vi "test-twist3d.vi"(8 "error in (no error)":errorcluster) -> (0 "error out":errorcluster, 3 "All PASSED":bool)   [LabVIEW 2019]
uses:
  <vilib>/Rock Robotics/WPI/ThirdParty/JAS_Junk/TrajLib/Pose3d_New_Trans3dRot3d.vi
  <vilib>/Rock Robotics/WPI/ThirdParty/JAS_Junk/TrajLib/Translation3d_Create_Default.vi
  <vilib>/Rock Robotics/WPI/ThirdParty/JAS_Junk/TrajLib/Quaternion_New_Default.vi
  <vilib>/Rock Robotics/WPI/ThirdParty/JAS_Junk/TrajLib/Quaternion_New.vi
  <vilib>/Rock Robotics/WPI/ThirdParty/JAS_Junk/TrajLib/Translation3d_Create.vi
  <vilib>/Rock Robotics/WPI/ThirdParty/JAS_Junk/TrajLib/Translation3d_Equals.vi
  <vilib>/Rock Robotics/WPI/ThirdParty/JAS_Junk/TrajLib/Rotation3d_Equals.vi
  <vilib>/Rock Robotics/WPI/ThirdParty/JAS_Junk/TrajLib/Pose3d_getTranslation3d.vi
  <vilib>/Rock Robotics/WPI/ThirdParty/JAS_Junk/TrajLib/Pose3d_getRotation3d.vi
  <vilib>/Rock Robotics/WPI/ThirdParty/JAS_Junk/TrajLib/Matrix_NormF.vi
  <vilib>/Rock Robotics/WPI/ThirdParty/JAS_Junk/TrajLib/Rotation3d_GetQuaterion.vi
  <vilib>/Rock Robotics/WPI/ThirdParty/JAS_Junk/TrajLib/Quaternion_Equals.vi
  <vilib>/Analysis/_algsub.llb/Matrix Norm.vi
  <vilib>/Analysis/_algsub.llb/Real Matrix Norm.vi
  <vilib>/Analysis/Matrix/Numeric/Conversions/Array To Matrix.vi
  <vilib>/Analysis/Matrix/Numeric/Conversions/Array To Matrix - RA.vi
  <vilib>/Rock Robotics/WPI/ThirdParty/JAS_Junk/TrajLib/Trajectory_Library.lvlib
panel:
  # "Twist3d Test"
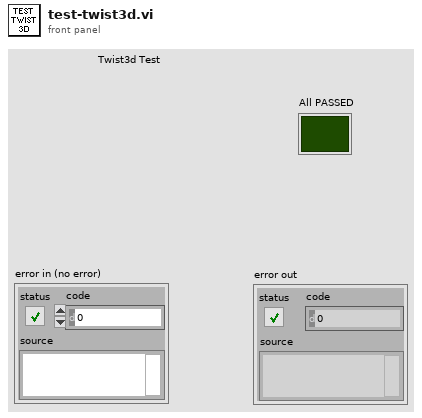
[diagram p1: front panel]
types:
  T1 = typedef "Trajectory_Library.lvlib/ROTATION3D.ctl" = cluster{"Q_quaternion":T2}
  T2 = typedef "Trajectory_Library.lvlib/QUATERNION.ctl" = cluster{"R":dbl, "V":dbl[]}
  T3 = typedef "Trajectory_Library.lvlib/POSE3D.ctl" = cluster{"Translation3d":T4, "Rotation3d":T1}
  T4 = typedef "Trajectory_Library.lvlib/TRANSLATION3D.ctl" = cluster{"X":dbl, "Y":dbl, "Z":dbl}
  T5 = typedef "Trajectory_Library.lvlib/TWIST3D.ctl" = cluster{"dX":dbl, "dY":dbl, "dZ":dbl, "rX":dbl, "rY":dbl, "rZ":dbl}
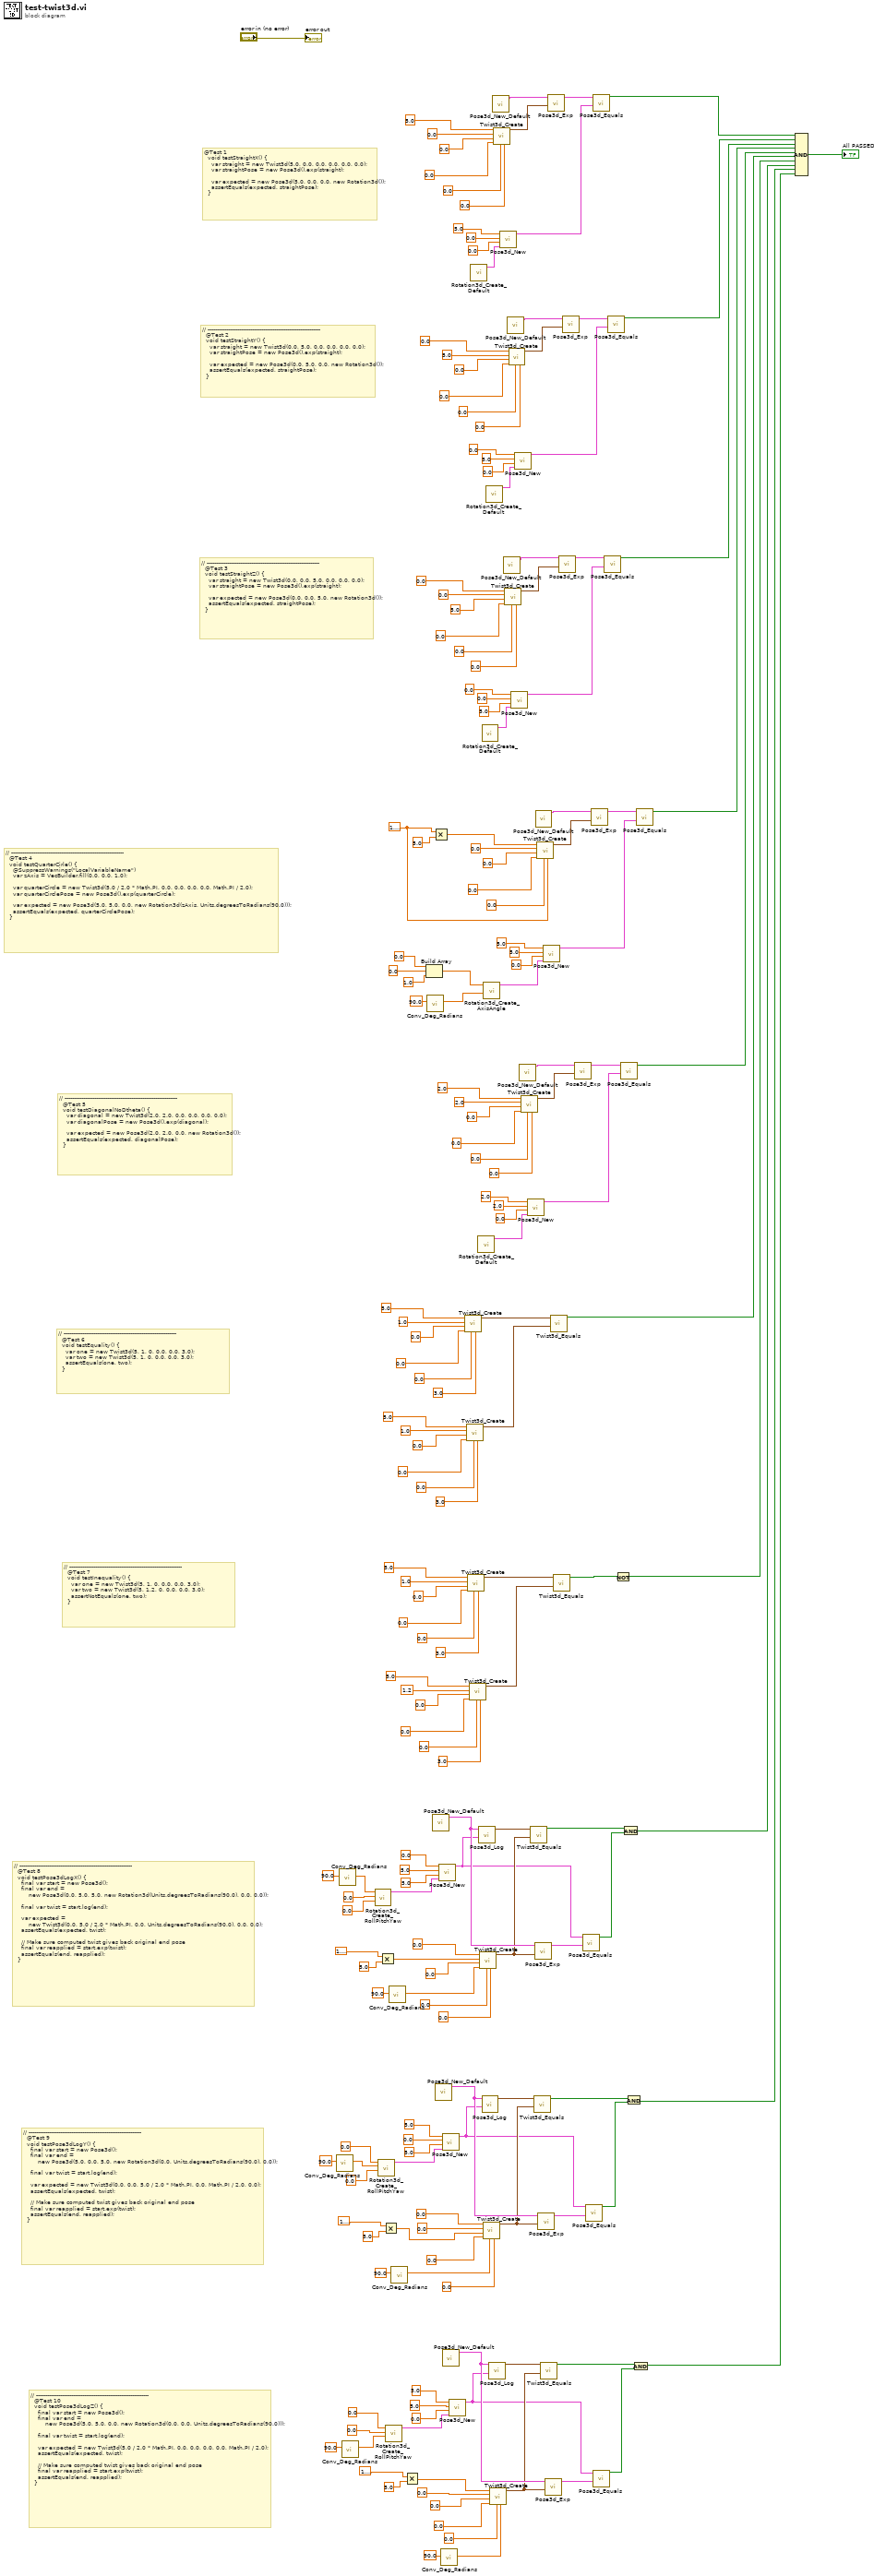
[diagram p0: block diagram]
diagram:
  w130 = 1.5707963267948966
  # "// -------------------------------------------------------------\n  @Test 10\n  void testPose3dLogZ() {\n    final var start = new Pose3d();\n    final var end =\n        new Pose3d(5.0, 5.0, 0.0, new Rotation3d(0.0, 0.0, Units.degreesToRadians(90.0)));\n\n    final var twist = start.log(end);\n\n    var expected = new Twist3d(5.0 / 2.0 * Math.PI, 0.0, 0.0, 0.0, 0.0, Math.PI / 2.0);\n    assertEquals(expected, twist);\n\n    // Make sure computed twist gives back original end pose\n    final var reapplied = start.exp(twist);\n    assertEquals(end, reapplied);\n  }"
  # "// -------------------------------------------------------------\n  @Test 9\n  void testPose3dLogY() {\n    final var start = new Pose3d();\n    final var end =\n        new Pose3d(5.0, 0.0, 5.0, new Rotation3d(0.0, Units.degreesToRadians(90.0), 0.0));\n\n    final var twist = start.log(end);\n\n    var expected = new Twist3d(0.0, 0.0, 5.0 / 2.0 * Math.PI, 0.0, Math.PI / 2.0, 0.0);\n    assertEquals(expected, twist);\n\n    // Make sure computed twist gives back original end pose\n    final var reapplied = start.exp(twist);\n    assertEquals(end, reapplied);\n  }"
  # "// -------------------------------------------------------------\n  @Test 8\n  void testPose3dLogX() {\n    final var start = new Pose3d();\n    final var end =\n        new Pose3d(0.0, 5.0, 5.0, new Rotation3d(Units.degreesToRadians(90.0), 0.0, 0.0));\n\n    final var twist = start.log(end);\n\n    var expected =\n        new Twist3d(0.0, 5.0 / 2.0 * Math.PI, 0.0, Units.degreesToRadians(90.0), 0.0, 0.0);\n    assertEquals(expected, twist);\n\n    // Make sure computed twist gives back original end pose\n    final var reapplied = start.exp(twist);\n    assertEquals(end, reapplied);\n  }"
  # "// -------------------------------------------------------------\n  @Test 7\n  void testInequality() {\n    var one = new Twist3d(5, 1, 0, 0.0, 0.0, 3.0);\n    var two = new Twist3d(5, 1.2, 0, 0.0, 0.0, 3.0);\n    assertNotEquals(one, two);\n  }"
  # "// -------------------------------------------------------------\n  @Test 6\n  void testEquality() {\n    var one = new Twist3d(5, 1, 0, 0.0, 0.0, 3.0);\n    var two = new Twist3d(5, 1, 0, 0.0, 0.0, 3.0);\n    assertEquals(one, two);\n  }"
  # "// -------------------------------------------------------------\n  @Test 5\n  void testDiagonalNoDtheta() {\n    var diagonal = new Twist3d(2.0, 2.0, 0.0, 0.0, 0.0, 0.0);\n    var diagonalPose = new Pose3d().exp(diagonal);\n\n    var expected = new Pose3d(2.0, 2.0, 0.0, new Rotation3d());\n    assertEquals(expected, diagonalPose);\n  }"
  # "// -------------------------------------------------------------\n  @Test 4\n  void testQuarterCirle() {\n    @SuppressWarnings(\"LocalVariableName\")\n    var zAxis = VecBuilder.fill(0.0, 0.0, 1.0);\n\n    var quarterCircle = new Twist3d(5.0 / 2.0 * Math.PI, 0.0, 0.0, 0.0, 0.0, Math.PI / 2.0);\n    var quarterCirclePose = new Pose3d().exp(quarterCircle);\n\n    var expected = new Pose3d(5.0, 5.0, 0.0, new Rotation3d(zAxis, Units.degreesToRadians(90.0)));\n    assertEquals(expected, quarterCirclePose);\n  }"
  # "// -------------------------------------------------------------\n  @Test 3\n  void testStraightZ() {\n    var straight = new Twist3d(0.0, 0.0, 5.0, 0.0, 0.0, 0.0);\n    var straightPose = new Pose3d().exp(straight);\n\n    var expected = new Pose3d(0.0, 0.0, 5.0, new Rotation3d());\n    assertEquals(expected, straightPose);\n  }"
  # "// -------------------------------------------------------------\n  @Test 2\n  void testStraightY() {\n    var straight = new Twist3d(0.0, 5.0, 0.0, 0.0, 0.0, 0.0);\n    var straightPose = new Pose3d().exp(straight);\n\n    var expected = new Pose3d(0.0, 5.0, 0.0, new Rotation3d());\n    assertEquals(expected, straightPose);\n  }"
  # "@Test 1\n  void testStraightX() {\n    var straight = new Twist3d(5.0, 0.0, 0.0, 0.0, 0.0, 0.0);\n    var straightPose = new Pose3d().exp(straight);\n\n    var expected = new Pose3d(5.0, 0.0, 0.0, new Rotation3d());\n    assertEquals(expected, straightPose);\n  }"
  n1 = call <vilib>:"Conv_Deg_Radians.vi"("Degress"=90.0) -> ("Radians"=w32:dbl)  [unwired: 10 in]
  n2 = call <vilib>:"Conv_Deg_Radians.vi"("Degress"=90.0) -> ("Radians"=w74:dbl)  [unwired: 10 in]
  n3 = call <vilib>:"Conv_Deg_Radians.vi"("Degress"=90.0) -> ("Radians"=w7:dbl)  [unwired: 10 in]
  n4 = call <vilib>:"Rotation3d_Create_RollPitchYaw.vi"("Yaw"=0.0, "Pitch"=0.0, "Roll"=w74) -> ("Rotation3d"=w71:T1)  [unwired: 8 in]
  n5 = call <vilib>:"Rotation3d_Create_RollPitchYaw.vi"("Yaw"=0.0, "Pitch"=w32, "Roll"=0.0 ("Pitch")) -> ("Rotation3d"=w48:T1)  [unwired: 8 in]
  n6 = Multiply(x=1.5707963267948966, y=5.0) -> (x*y=w62:dbl)
  n7 = Multiply(x=1.5707963267948966, y=5.0) -> (x*y=w29:dbl)
  n8 = call <vilib>:"Rotation3d_Create_RollPitchYaw.vi"("Yaw"=w7, "Pitch"=0.0 ("Yaw"), "Roll"=0.0 ("Pitch")) -> ("Rotation3d"=w24:T1)  [unwired: 8 in]
  n9 = call <vilib>:"Conv_Deg_Radians.vi"("Degress"=90.0) -> ("Radians"=w60:dbl)  [unwired: 10 in]
  n10 = call <vilib>:"Conv_Deg_Radians.vi"("Degress"=90.0) -> ("Radians"=w27:dbl)  [unwired: 10 in]
  n11 = Multiply(x=1.5707963267948966, y=5.0) -> (x*y=w6:dbl)
  n12 = Build Array(0.0 ("element"), 0.0 ("element"), 1.0 ("element")) -> (w128:dbl[])
  n13 = call <vilib>:"Conv_Deg_Radians.vi"("Degress"=90.0) -> ("Radians"=w126:dbl)  [unwired: 10 in]
  n14 = call <vilib>:"Pose3d_New_Default.vi"() -> ("outPose3d"=w57:T3)  [unwired: 11 in]
  n15 = Multiply(x=w130, y=5.0) -> (x*y=w131:dbl)
  n16 = call <vilib>:"Pose3d_New_Default.vi"() -> ("outPose3d"=w38:T3)  [unwired: 11 in]
  n17 = call <vilib>:"Pose3d_New.vi"("Rotation3d"=w71, "z"=5.0, "Y"=5.0, "X"=0.0) -> ("out Pose3d"=w55:T3)  [unwired: 7 in]
  n18 = call <vilib>:"Conv_Deg_Radians.vi"("Degress"=90.0) -> ("Radians"=w2:dbl)  [unwired: 10 in]
  n19 = call <vilib>:"Pose3d_New.vi"("Rotation3d"=w48, "z"=5.0, "Y"=0.0, "X"=5.0) -> ("out Pose3d"=w36:T3)  [unwired: 7 in]
  n20 = call <vilib>:"Pose3d_New_Default.vi"() -> ("outPose3d"=w16:T3)  [unwired: 11 in]
  n21 = call <vilib>:"Pose3d_New.vi"("Rotation3d"=w24, "z"=0.0, "Y"=5.0, "X"=5.0) -> ("out Pose3d"=w14:T3)  [unwired: 7 in]
  n22 = call <vilib>:"Twist3d_Create.vi"("rZ"=3.0 ("y"), "rY"=0.0, "rX"=0.0, "dZ"=0.0, "dY"=1.0, "dX"=5.0) -> ("Twist3d"=w94:T5)  [unwired: 5 in]
  n23 = call <vilib>:"Twist3d_Create.vi"("rZ"=3.0 ("y"), "rY"=0.0, "rX"=0.0, "dZ"=0.0, "dY"=1.0, "dX"=5.0) -> ("Twist3d"=w93:T5)  [unwired: 5 in]
  n24 = call <vilib>:"Twist3d_Create.vi"("rZ"=3.0 ("y"), "rY"=0.0, "rX"=0.0, "dZ"=0.0, "dY"=1.0, "dX"=5.0) -> ("Twist3d"=w79:T5)  [unwired: 5 in]
  n25 = call <vilib>:"Twist3d_Create.vi"("rZ"=3.0 ("y"), "rY"=0.0, "rX"=0.0, "dZ"=0.0, "dY"=1.2, "dX"=5.0) -> ("Twist3d"=w78:T5)  [unwired: 5 in]
  n26 = call <vilib>:"Rotation3d_Create_Default.vi"() -> ("ROTATION3D"=w180:T1)  [unwired: 11 in]
  n27 = call <vilib>:"Rotation3d_Create_Default.vi"() -> ("ROTATION3D"=w109:T1)  [unwired: 11 in]
  n28 = call <vilib>:"Pose3d_Log.vi"("end Pose3d"=w55, "in Pose3d"=w57) -> ("out Twist3d"=w58:T5)  [unwired: 9 in]
  n29 = call <vilib>:"Twist3d_Create.vi"("rZ"=0.0 ("rY"), "rY"=0.0, "rX"=w60, "dZ"=0.0, "dY"=w62, "dX"=0.0 ("dY")) -> ("Twist3d"=w56:T5)  [unwired: 5 in]
  n30 = call <vilib>:"Rotation3d_Create_Default.vi"() -> ("ROTATION3D"=w150:T1)  [unwired: 11 in]
  n31 = call <vilib>:"Pose3d_Log.vi"("end Pose3d"=w36, "in Pose3d"=w38) -> ("out Twist3d"=w39:T5)  [unwired: 9 in]
  n32 = call <vilib>:"Twist3d_Create.vi"("rZ"=0.0 ("rY"), "rY"=w27, "rX"=0.0 ("rY"), "dZ"=w29, "dY"=0.0 ("dZ"), "dX"=0.0 ("dY")) -> ("Twist3d"=w37:T5)  [unwired: 5 in]
  n33 = call <vilib>:"Rotation3d_Create_AxisAngle.vi"("Angle"=w126, "Axis Vector"=w128) -> ("Rotation3d"=w125:T1)  [unwired: 9 in]
  n34 = call <vilib>:"Rotation3d_Create_Default.vi"() -> ("ROTATION3D"=w165:T1)  [unwired: 11 in]
  n35 = call <vilib>:"Pose3d_Log.vi"("end Pose3d"=w14, "in Pose3d"=w16) -> ("out Twist3d"=w17:T5)  [unwired: 9 in]
  n36 = call <vilib>:"Twist3d_Create.vi"("rZ"=w2, "rY"=0.0, "rX"=0.0 ("rY"), "dZ"=0.0 ("dY"), "dY"=0.0 ("dZ"), "dX"=w6) -> ("Twist3d"=w15:T5)  [unwired: 5 in]
  n37 = call <vilib>:"Pose3d_New_Default.vi"() -> ("outPose3d"=w182:T3)  [unwired: 11 in]
  n38 = call <vilib>:"Twist3d_Create.vi"("rZ"=0.0, "rY"=0.0, "rX"=0.0, "dZ"=0.0, "dY"=0.0, "dX"=5.0) -> ("Twist3d"=w181:T5)  [unwired: 5 in]
  n39 = call <vilib>:"Pose3d_New.vi"("Rotation3d"=w180, "z"=0.0, "Y"=0.0, "X"=5.0) -> ("out Pose3d"=w175:T3)  [unwired: 7 in]
  n40 = call <vilib>:"Pose3d_New_Default.vi"() -> ("outPose3d"=w152:T3)  [unwired: 11 in]
  n41 = call <vilib>:"Twist3d_Create.vi"("rZ"=0.0, "rY"=0.0, "rX"=0.0, "dZ"=5.0, "dY"=0.0, "dX"=0.0) -> ("Twist3d"=w151:T5)  [unwired: 5 in]
  n42 = call <vilib>:"Pose3d_New_Default.vi"() -> ("outPose3d"=w167:T3)  [unwired: 11 in]
  n43 = call <vilib>:"Twist3d_Create.vi"("rZ"=0.0, "rY"=0.0, "rX"=0.0, "dZ"=0.0, "dY"=5.0, "dX"=0.0) -> ("Twist3d"=w166:T5)  [unwired: 5 in]
  n44 = call <vilib>:"Pose3d_New.vi"("Rotation3d"=w150, "z"=5.0, "Y"=0.0, "X"=0.0) -> ("out Pose3d"=w145:T3)  [unwired: 7 in]
  n45 = call <vilib>:"Pose3d_New.vi"("Rotation3d"=w165, "z"=0.0, "Y"=5.0, "X"=0.0) -> ("out Pose3d"=w160:T3)  [unwired: 7 in]
  n46 = call <vilib>:"Pose3d_New_Default.vi"() -> ("outPose3d"=w117:T3)  [unwired: 11 in]
  n47 = call <vilib>:"Twist3d_Create.vi"("rZ"=0.0 ("y"), "rY"=0.0, "rX"=0.0, "dZ"=0.0, "dY"=2.0, "dX"=2.0) -> ("Twist3d"=w116:T5)  [unwired: 5 in]
  n48 = call <vilib>:"Pose3d_New.vi"("Rotation3d"=w109, "z"=0.0, "Y"=2.0, "X"=2.0) -> ("out Pose3d"=w111:T3)  [unwired: 7 in]
  n49 = call <vilib>:"Twist3d_Equals.vi"("other Twist3d"=w56, "this Twist3d"=w58) -> ("Equals"=w53:bool)  [unwired: 9 in]
  n50 = call <vilib>:"Twist3d_Equals.vi"("other Twist3d"=w37, "this Twist3d"=w39) -> ("Equals"=w34:bool)  [unwired: 9 in]
  n51 = call <vilib>:"Pose3d_Exp.vi"("Twist3d"=w56, "Pose3d"=w57) -> ("Updated Pose3d"=w54:T3)  [unwired: 9 in]
  n52 = call <vilib>:"Pose3d_New_Default.vi"() -> ("outPose3d"=w139:T3)  [unwired: 11 in]
  n53 = call <vilib>:"Twist3d_Create.vi"("rZ"=w130, "rY"=0.0, "rX"=0.0, "dZ"=0.0, "dY"=0.0, "dX"=w131) -> ("Twist3d"=w138:T5)  [unwired: 5 in]
  n54 = call <vilib>:"Pose3d_Exp.vi"("Twist3d"=w37, "Pose3d"=w38) -> ("Updated Pose3d"=w35:T3)  [unwired: 9 in]
  n55 = call <vilib>:"Twist3d_Equals.vi"("other Twist3d"=w15, "this Twist3d"=w17) -> ("Equals"=w12:bool)  [unwired: 9 in]
  n56 = call <vilib>:"Pose3d_New.vi"("Rotation3d"=w125, "z"=0.0, "Y"=5.0, "X"=5.0) -> ("out Pose3d"=w133:T3)  [unwired: 7 in]
  n57 = call <vilib>:"Pose3d_Exp.vi"("Twist3d"=w15, "Pose3d"=w16) -> ("Updated Pose3d"=w13:T3)  [unwired: 9 in]
  n58 = call <vilib>:"Pose3d_Exp.vi"("Twist3d"=w181, "Pose3d"=w182) -> ("Updated Pose3d"=w176:T3)  [unwired: 9 in]
  n59 = call <vilib>:"Twist3d_Equals.vi"("other Twist3d"=w93, "this Twist3d"=w94) -> ("Equals"=w92:bool)  [unwired: 9 in]
  n60 = call <vilib>:"Twist3d_Equals.vi"("other Twist3d"=w78, "this Twist3d"=w79) -> ("Equals"=w76:bool)  [unwired: 9 in]
  n61 = call <vilib>:"Pose3d_Exp.vi"("Twist3d"=w151, "Pose3d"=w152) -> ("Updated Pose3d"=w146:T3)  [unwired: 9 in]
  n62 = call <vilib>:"Pose3d_Exp.vi"("Twist3d"=w166, "Pose3d"=w167) -> ("Updated Pose3d"=w161:T3)  [unwired: 9 in]
  n63 = call <vilib>:"Pose3d_Exp.vi"("Twist3d"=w116, "Pose3d"=w117) -> ("Updated Pose3d"=w112:T3)  [unwired: 9 in]
  n64 = call <vilib>:"Pose3d_Equals.vi"("other Pose3d"=w54, "in Pose3d"=w55) -> ("Equals"=w52:bool)  [unwired: 9 in]
  n65 = call <vilib>:"Pose3d_Equals.vi"("other Pose3d"=w35, "in Pose3d"=w36) -> ("Equals"=w33:bool)  [unwired: 9 in]
  n66 = call <vilib>:"Pose3d_Exp.vi"("Twist3d"=w138, "Pose3d"=w139) -> ("Updated Pose3d"=w134:T3)  [unwired: 9 in]
  n67 = call <vilib>:"Pose3d_Equals.vi"("other Pose3d"=w13, "in Pose3d"=w14) -> ("Equals"=w11:bool)  [unwired: 9 in]
  n68 = call <vilib>:"Pose3d_Equals.vi"("other Pose3d"=w175, "in Pose3d"=w176) -> ("Equals"=w174:bool)  [unwired: 9 in]
  n69 = call <vilib>:"Pose3d_Equals.vi"("other Pose3d"=w145, "in Pose3d"=w146) -> ("Equals"=w144:bool)  [unwired: 9 in]
  n70 = call <vilib>:"Pose3d_Equals.vi"("other Pose3d"=w160, "in Pose3d"=w161) -> ("Equals"=w159:bool)  [unwired: 9 in]
  n71 = Not(x=w76) -> (.not. x?=w77:bool)
  n72 = call <vilib>:"Pose3d_Equals.vi"("other Pose3d"=w111, "in Pose3d"=w112) -> ("Equals"=w107:bool)  [unwired: 9 in]
  n73 = And(x=w53, y=w52) -> (x .and. y?=w51:bool)
  n74 = And(x=w34, y=w33) -> (x .and. y?=w26:bool)
  n75 = And(x=w12, y=w11) -> (x .and. y?=w1:bool)
  n76 = call <vilib>:"Pose3d_Equals.vi"("other Pose3d"=w133, "in Pose3d"=w134) -> ("Equals"=w122:bool)  [unwired: 9 in]
  n77 = Compound Arithmetic op=AND(w174, w159, w144, w122, w107, w92, w77, w51, w26, w1) -> (→"All PASSED":bool)
  "error out" <- "error in (no error)"
